vi "GetStatusWord.vi"(8 "error in (no error)":errorcluster, 11 "Motor Base in":refnum<class "Motor Base.lvclass">) -> (0 "error out":errorcluster, 2 "Fault":bool, 3 "Motor Base out":refnum<class "Motor Base.lvclass">)   [LabVIEW 2016, in "Motor Base.lvlib" / "Motor Base.lvclass"]
uses:
  Motor Base.lvclass
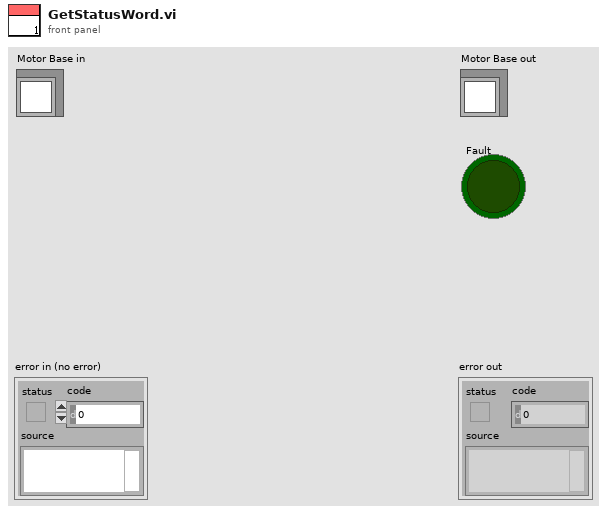
[diagram p1: front panel]
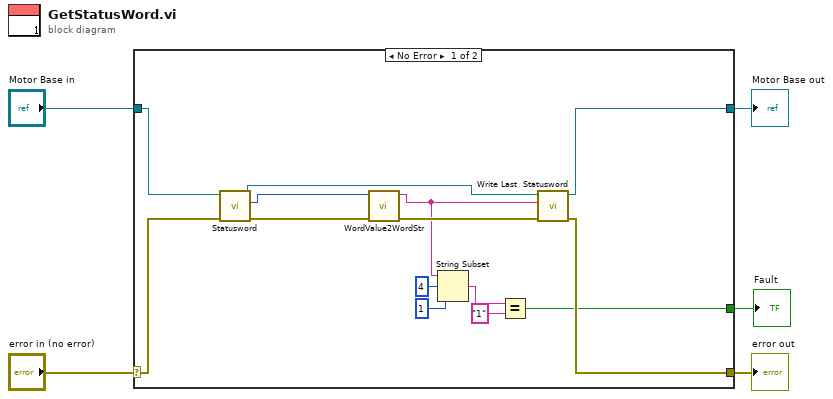
[diagram p0: block diagram]
diagram:
  n1 = case shown="No Error" "error in (no error)" {
    selector: "error in (no error)" -> [w18 w21]
    tunnel: [w13 w21] -> w4
    tunnel: [w12 w20] -> w2
    tunnel: "Motor Base in" -> [w19 w20]
    tunnel: [w7 _] -> w1
    frame No Error {
      n2 = call-dynamic "Statusword.vi"("error in"=w18, "Motor Base in"=w19) -> ("error out"=w16:errorcluster, "Data"=w14:i64, "Motor Base out"=w17:refnum<class "Motor Base.lvclass">)  [unwired: 7 in]
      n3 = call "WordValue2WordStr.vi"("error in"=w16, "WordValue"=w14) -> ("error out"=w15:errorcluster, "WordStr"=w6:string)  [unwired: 8 in]
      n4 = String Subset(string=w6, offset (0)=4, length (rest)=1 ("length (rest)")) -> (substring=w9:string)
      n5 = Equal?(x=w9, y="1") -> (x = y?=w7:bool)
      n6 = call-dynamic "Write Last  Statusword.vi"("error in (no error)"=w15, "Statusword"=w6, "Motor Base in"=w17) -> ("error out"=w13:errorcluster, "Motor Base out"=w12:refnum<class "Motor Base.lvclass">)  [unwired: 7 in]
    }
    frame Error {
    }
  }
  "error out" <- w4
  "Motor Base out" <- w2
  "Fault" <- w1
